vi "GetDeviceInfo.vi"(8 "error in (no error)":errorcluster, 11 "Device In":u64) -> (0 "error out":errorcluster, 1 "ChannelClassName":string, 2 "Device Info":T1={"Serial Number"=-1, "Channel"=0, "Port"=0}, 3 "Device Out":u64, 4 "Connection":u16(ring) items=["No Preference", "Remote", "Local"], 5 "Channel Class":u32(ring) items=["PHIDCHCLASS_NOTHING", "PHIDCHCLASS_ACCELEROMETER", "PHIDCHCLASS_CURRENTINPUT", "PHIDCHCLASS_DATAADAPTER", "PHIDCHCLASS_DCMOTOR", "PHIDCHCLASS_DIGITALINPUT", "PHIDCHCLASS_DIGITALOUTPUT", "PHIDCHCLASS_DISTANCESENSOR", "PHIDCHCLASS_ENCODER", "PHIDCHCLASS_FREQUENCYCOUNTER", "PHIDCHCLASS_GPS", "PHIDCHCLASS_LCD", "PHIDCHCLASS_GYROSCOPE", "PHIDCHCLASS_HUB", "PHIDCHCLASS_HUMANINPUT", "PHIDCHCLASS_HUMIDITYSENSOR", "PHIDCHCLASS_IR", "PHIDCHCLASS_LIGHTSENSOR", "PHIDCHCLASS_MAGNETOMETER", "PHIDCHCLASS_MESHDONGLE", "PHIDCHCLASS_POWERGUARD", "PHIDCHCLASS_PRESSURESENSOR", "PHIDCHCLASS_RCSERVO", "PHIDCHCLASS_RESISTANCEINPUT", "PHIDCHCLASS_RFID", "PHIDCHCLASS_SOUNDSENSOR", "PHIDCHCLASS_SPATIAL", "PHIDCHCLASS_STEPPER", "PHIDCHCLASS_TEMPERATURESENSOR", "PHIDCHCLASS_VOLTAGEINPUT", "PHIDCHCLASS_VOLTAGEOUTPUT", "PHIDCHCLASS_VOLTAGERATIOINPUT", "", "", "PHIDCHCLASS_MOTORPOSITIONCONTROLLER", "PHIDCHCLASS_BLDCMOTOR", "PHIDCHCLASS_DICTIONARY"])   [LabVIEW 2012, in "Phidget Common.lvlib"]
doc: "Gets all device information required to open a Phidget channel. Intended for use to open a Phidget after it has been discovered by the Phidget Manager."
uses:
  <instrlib>/Phidgets/Phidget Common/Phidget Common.lvlib
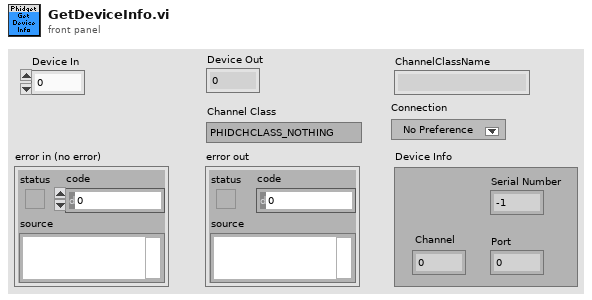
[diagram p1: front panel]
types:
  T1 = cluster{"Serial Number":i32, "Channel":i32, "Port":i32}
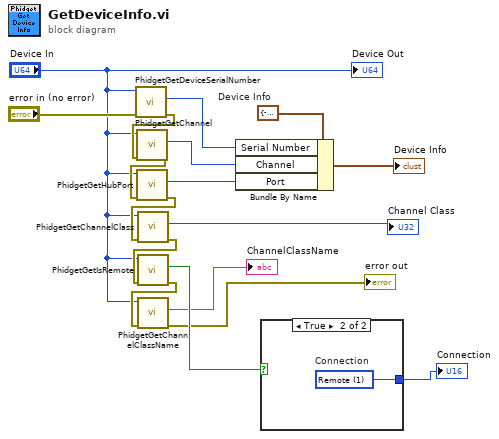
[diagram p0: block diagram]
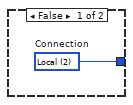
[diagram p2: hidden frame]
diagram:
  w17 = T1 {"Serial Number"=-1, "Channel"=0, "Port"=0}  # Device Info
  n1 = call <instrlib>:"PhidgetGetDeviceSerialNumber.vi"("error in"="error in (no error)", "Device In"="Device In") -> ("error out"=w13:errorcluster, "SerialNumber"=w16:i32)  [unwired: 7 in, 1 out]
  n2 = call <instrlib>:"PhidgetGetChannel.vi"("error in (no error)"=w13, "Device In"="Device In") -> ("error out"=w12:errorcluster, "Channel"=w15:i32)  [unwired: 6 in, 1 out]
  n3 = call <instrlib>:"PhidgetGetHubPort.vi"("error in"=w12, "Device In"="Device In") -> ("error out"=w9:errorcluster, "Hub Port"=w14:i32)  [unwired: 7 in, 1 out]
  n4 = call <instrlib>:"PhidgetGetChannelClass.vi"("error in (no error)"=w9, "Device In"="Device In") -> ("error out"=w7:errorcluster, "Channel Class"=→"Channel Class":u32)  [unwired: 6 in, 1 out]
  n5 = call <instrlib>:"PhidgetGetIsRemote.vi"("error in (no error)"=w7, "Device In"="Device In") -> ("error out"=w4:errorcluster, "Remote"=w6:bool)  [unwired: 6 in, 1 out]
  n6 = call <instrlib>:"PhidgetGetChannelClassName.vi"("error in"=w4, "Device In"="Device In") -> ("error out"=→"error out":errorcluster, "ChannelClassName"=→"ChannelClassName":string)  [unwired: 7 in, 1 out]
  n7 = Bundle By Name(cluster=w17, "Serial Number"=w16, "Channel"=w15, "Port"=w14) -> (→"Device Info":T1)
  n8 = case shown="True" w6 {
    tunnel: [w18 w19] -> w5
    frame False {
      w18 = u16 2 items=["No Preference", "Remote", "Local"]  # Connection
    }
    frame True {
      w19 = u16 1 items=["No Preference", "Remote", "Local"]  # Connection
    }
  }
  "Connection" <- w5
  "Device Out" <- "Device In"
